vi "Results (Dictionary) to X and Y Arrays.vi"(11 "Results (Dictionary)":cluster{"key":string, "value":dbl}[](array[cluster])) -> (2 "Y":dbl[](array[numeric]), 3 "X":dbl[](array[numeric]))   [LabVIEW 2019, in "Transport.lvclass"]
uses:
  Transport.lvclass
  <userlib>/LevyLab/Lockin-Multichannel/Instrument.Lockin/Typedefs/Results Type--Enum.ctl
  <userlib>/LevyLab/Lockin-Multichannel/Instrument.Lockin/Instrument.Lockin.lvclass
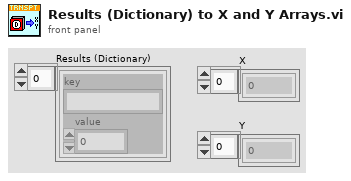
[diagram p1: front panel]
types:
  T1 = typedef "Instrument.Lockin.lvlib/Instrument.Lockin.lvclass/Results Type--Enum.ctl" = enum16{"X", "Y", "R", "Theta", "Mean"}
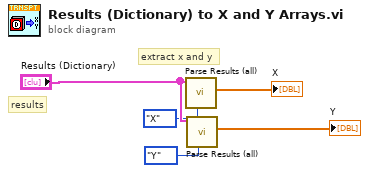
[diagram p0: block diagram]
diagram:
  # "extract x and y"
  # "results"
  n1 = call <userlib>:"Parse Results (all).vi"("Type"=Results_Type--Enum."X", "Results (Dictionary)"="Results (Dictionary)") -> ("Data"=→"X":dbl[])  [unwired: 6 in, 3 out]
  n2 = call <userlib>:"Parse Results (all).vi"("Type"=Results_Type--Enum."Y", "Results (Dictionary)"="Results (Dictionary)") -> ("Data"=→"Y":dbl[])  [unwired: 6 in, 3 out]
